vi "generate file string.vi"(8 "error in":errorcluster, 11 "file format":T1) -> (0 "error out":errorcluster, 3 "data string":string)   [LabVIEW 2013, in "PLConfigurationSerializer.lvlib"]
uses:
  PLConfigurationSerializer.lvlib
  file format.ctl
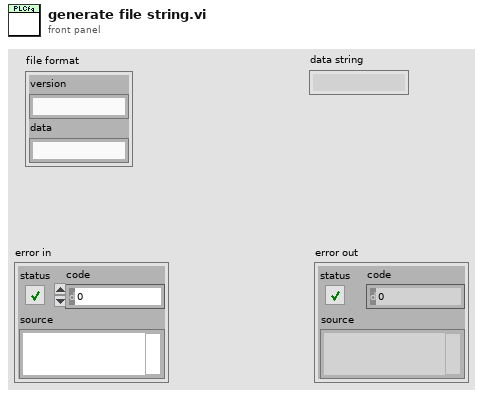
[diagram p1: front panel]
types:
  T1 = typedef "PLConfigurationSerializer.lvlib/file format.ctl" = cluster{"version":string, "data":string}
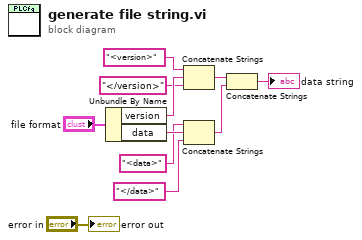
[diagram p0: block diagram]
diagram:
  n1 = Unbundle By Name("file format") -> ("version"=w10:string, "data"=w9:string)
  n2 = Concatenate Strings("<version>" ("identifier"), w10, "</version>" ("identifier")) -> (w5:string)
  n3 = Concatenate Strings("<data>" ("string"), w9, "</data>" ("string")) -> (w8:string)
  n4 = Concatenate Strings(w5, w8) -> (→"data string":string)
  "error out" <- "error in"
